vi "Register Events.vi"(8 "error in":errorcluster, 11 "XML Editor GUI in":refnum<class "XML Editor GUI.lvclass">) -> (0 "error out":errorcluster, 3 "XML Editor GUI out":refnum<class "XML Editor GUI.lvclass">, 4 "user event out":refnum<user-event>, 5 "Event Registration Refnum":refnum<event-registration>)   [LabVIEW 2014, in "XML Editor GUI.lvclass"]
uses:
  XML Editor GUI.lvclass
panel:
  in  "error in 2":errorcluster
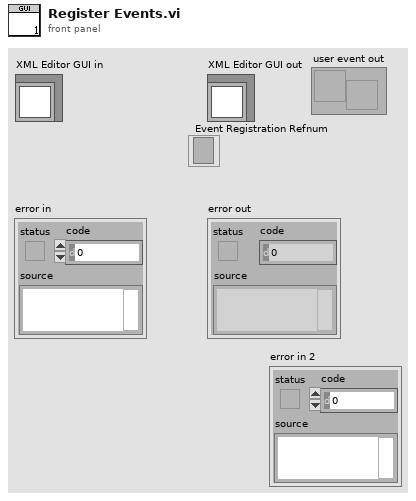
[diagram p1: front panel]
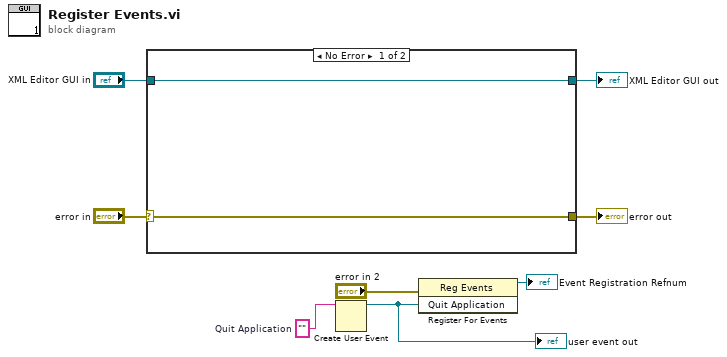
[diagram p0: block diagram]
diagram:
  w4 = ""  # Quit Application
  n1 = case shown="No Error" "error in" {
    selector: "error in" -> [w9 w12]
    tunnel: [w9 w12] -> w7
    tunnel: [w10 w11] -> w5
    tunnel: "XML Editor GUI in" -> [w10 w11]
    frame No Error {
    }
    frame Error {
    }
  }
  "error out" <- w7
  "XML Editor GUI out" <- w5
  n2 = Create User Event(user event datatype=w4) -> (user event=w2:refnum<user-event>)  [unwired: 1 in, 1 out]
  "user event out" <- w2
  n3 = register-events(error in="error in 2", w2) -> (reference out=→"Event Registration Refnum":refnum<event-registration>)  [unwired: 1 in, 1 out]
